vi "Get Error Definitions.vi"(9 "Deploy Errors?":bool) -> (2 "Err Defs":T1(array[cluster]), 3 "Unique Paths":string[](array[string]))   [LabVIEW 2014, in "PL Framework Configuration Tool.lvlib"]
uses:
  PL Framework Configuration Tool.lvlib
  <vilib>/NI/RT Management/classes/File Transfer Behavior/File Transfer Behavior.lvclass
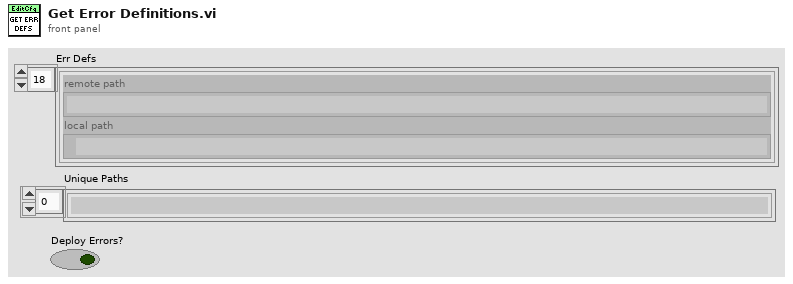
[diagram p1: front panel]
types:
  T1 = cluster{"remote path":string, "local path":path}[]
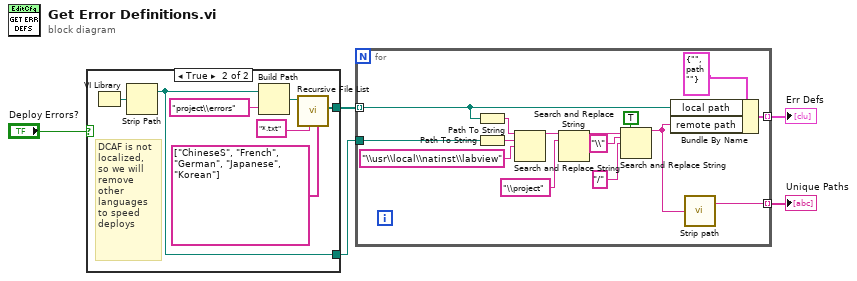
[diagram p0: block diagram]
diagram:
  n1 = case shown="True" "Deploy Errors?" {
    tunnel: [_ w10] -> w5
    tunnel: [_ w7] -> w4
    frame False {
    }
    frame True {
      # "DCAF is not\nlocalized,\nso we will\nremove \nother \nlanguages\nto speed \ndeploys"
      n2 = VI Library() -> (path=w8:path)
      n3 = Strip Path(path=w8) -> (stripped path=w7:path)  [unwired: 1 out]
      n4 = Build Path(base path=w7, name or relative path="project\\errors") -> (appended path=w9:path)
      n5 = call <vilib>:"Recursive File List.vi"("Folders to Exclude"=string[] ["ChineseS", "French", "German", "Japanese", "Korean"], "pattern"="*.txt", "Folder Path"=w9) -> ("All Files in Dir"=w10:path[])  [unwired: 4 in, 4 out]
    }
  }
  n6 = for {
    tunnel: w5 -> [w24] mode=indexing
    tunnel: w4 -> [w27]
    tunnel: [w23] -> w2 mode=indexing
    tunnel: [w21] -> w1 mode=indexing
    n7 = Path To String(path=w24) -> (string=w26:string)
    n8 = Path To String(path=w27) -> (string=w25:string)
    n9 = Search and Replace String(input string=w26, search string=w25, replace string="\\usr\\local\\natinst\\labview" ("replace string (\"\")")) -> (result string=w15:string)  [unwired: 5 in, 3 out]
    n10 = Search and Replace String(input string=w15, search string="\\project") -> (result string=w14:string)  [unwired: 6 in, 3 out]
    n11 = Search and Replace String(replace all?=TRUE ("replace all? (F)"), input string=w14, search string="\\", replace string="/" ("replace string (\"\")")) -> (result string=w17:string)  [unwired: 4 in, 3 out]
    n12 = Bundle By Name(cluster=cluster{"remote path":string, "local path":path} {"remote path"="", "local path"=path ""} ("transfer spec"), "local path"=w24, "remote path"=w17) -> (w23:cluster{"remote path":string, "local path":path})
    n13 = call <vilib>:"Strip path.vi"("Path"=w17) -> ("Stripped path"=w21:string)  [unwired: 2 in, 1 out]
  }
  "Err Defs" <- w2
  "Unique Paths" <- w1
